vi "QCP_TuningModeGet.vi"(8 "error in (no error)":errorcluster, 11 "QCP_DevRef_In":T1) -> (0 "error out":errorcluster, 2 "Tuning":bool, 3 "QCP_DevRef_Out":T1)   [LabVIEW 2016]
uses:
  <userlib>/836-libraries/System/QCP_V2/QCPSupportCode/QCP_RefNum.ctl
  <userlib>/836-libraries/System/QCP_V2/QCPSupportCode/QCPData.ctl
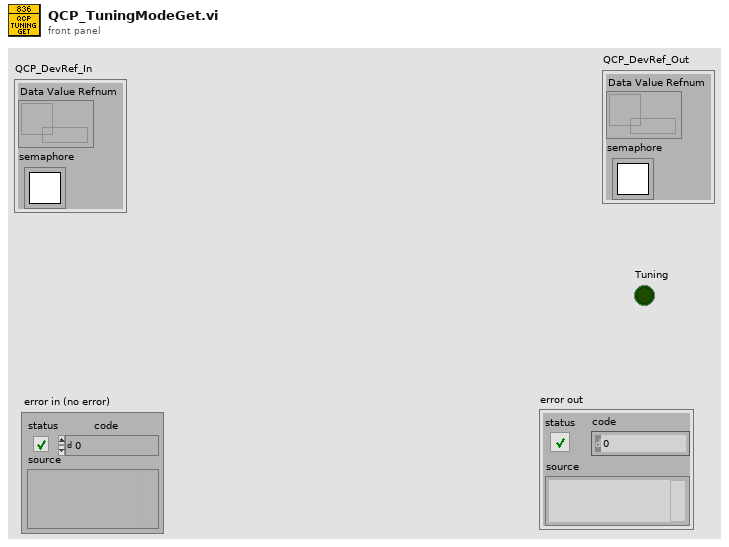
[diagram p1: front panel]
types:
  T1 = typedef "QCP_RefNum.ctl" = cluster{"Data Value Refnum":refnum<data-value>, "semaphore":T2}
  T2 = typedef "Semaphore RefNum" = refnum<k1>
  T3 = typedef "QCPData.ctl" = cluster{"Names":string[], "Values":cluster{"Array":dbl[]}[], "TuningMode?":bool}
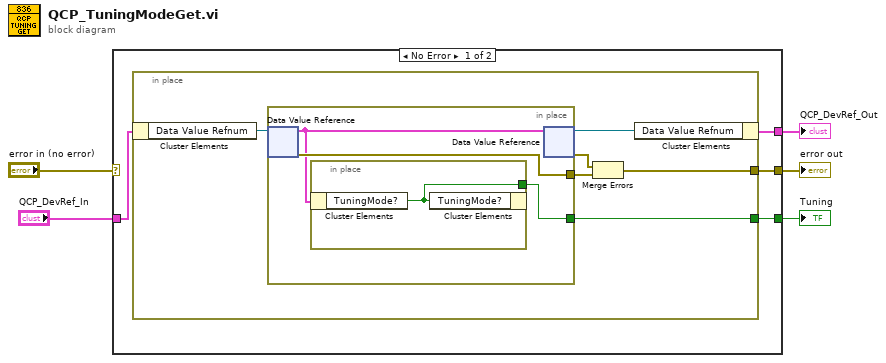
[diagram p0: block diagram]
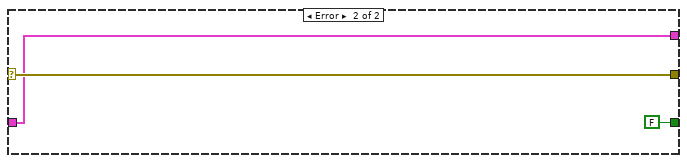
[diagram p2: hidden frame]
diagram:
  n1 = case shown="No Error" "error in (no error)" {
    selector: "error in (no error)" -> [_ w22]
    tunnel: [w9 FALSE ("TuningMode?")] -> w4
    tunnel: [w8 w22] -> w3
    tunnel: [w7 w21] -> w2
    tunnel: "QCP_DevRef_In" -> [w6 w21]
    frame No Error {
      n2 = in-place {
        in-place-border: [w11] -> w9
        in-place-border: [w10] -> w8
        n3 = in-place-cluster #1(w6) -> ("Data Value Refnum"=w15:refnum<data-value>)
        n4 = in-place {
          in-place-border: [w18] -> w13
          in-place-border: [w17] -> w11
          n5 = in-place-dvr #2(w15) -> (w16:T3, w18:errorcluster)
          n6 = in-place {
            in-place-border: [w19] -> w17
            n7 = in-place-cluster #3(w16) -> ("TuningMode?"=w19:bool)
            n8 = in-place-cluster #3("TuningMode?"=w19) -> ()  [unwired: 1 out]
          }
          n9 = in-place-dvr #2(w16) -> (w14:refnum<data-value>, w12:errorcluster)
        }
        n10 = Merge Errors(w12, w13) -> (w10:errorcluster)
        n11 = in-place-cluster #1("Data Value Refnum"=w14) -> (w7:T1)
      }
    }
    frame Error {
    }
  }
  "error out" <- w3
  "QCP_DevRef_Out" <- w2
  "Tuning" <- w4
